vi "Timing FGV.vi"(8 "error in (no error)":errorcluster, 9 "Target time (s)":dbl format="%#_13g", 10 "Index":i32, 11 "Method (Get Time)":enum16{"Start", "Stop", "Reset", "Get Time"}(ring)=enum."Get Time") -> (0 "error out":errorcluster, 2 "Done":bool, 3 "Time Remaining(s)":dbl)   [LabVIEW 2013]
panel:
  out "Running":bool
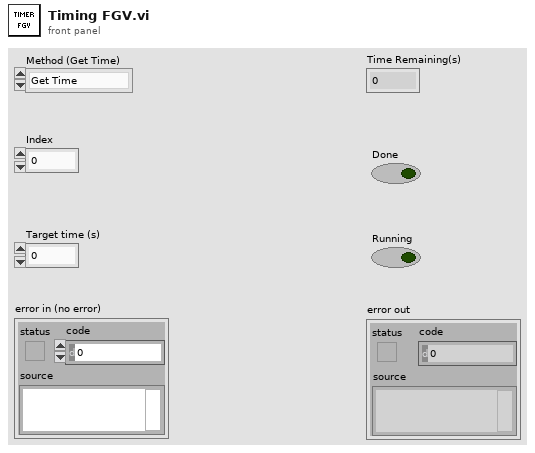
[diagram p1: front panel]
types:
  T1 = cluster{"Start Time":dbl, "Time Remaining":dbl, "Running":bool, "Done":bool}
  T2 = cluster{"Start Time":dbl, "Time Remaining":dbl, "Running":bool, "Done":bool}[]
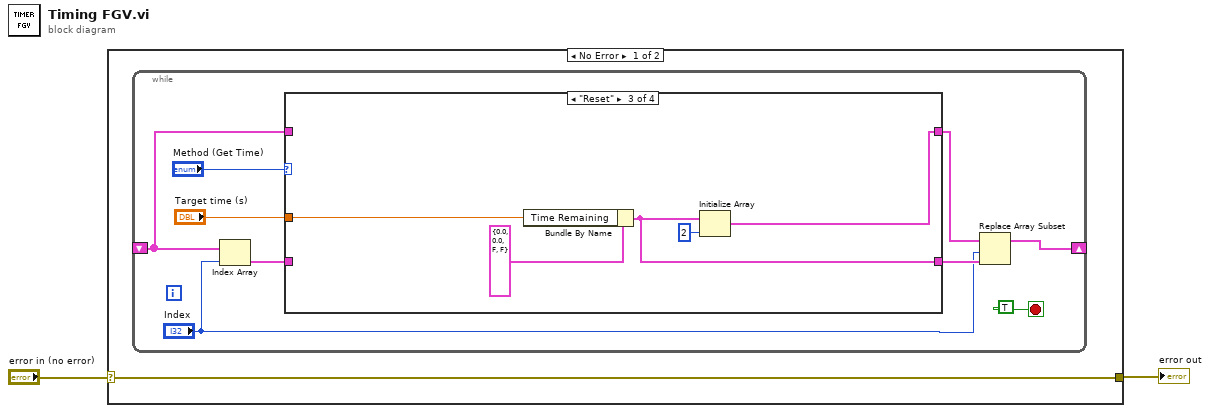
[diagram p0: block diagram]
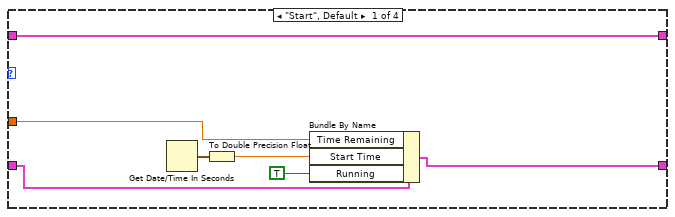
[diagram p2: hidden frame]
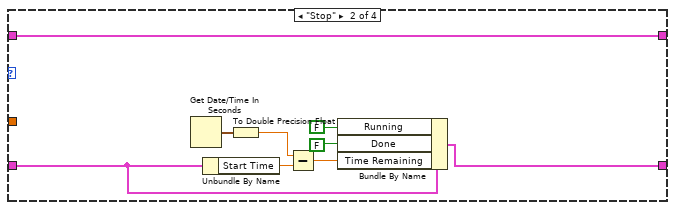
[diagram p3: hidden frame]
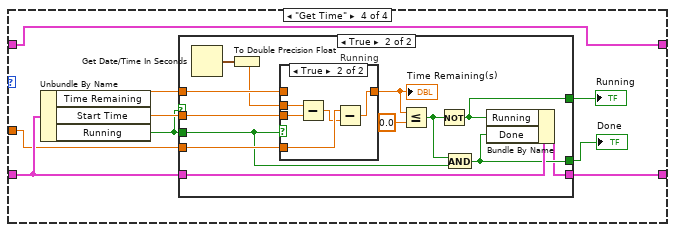
[diagram p4: hidden frame]
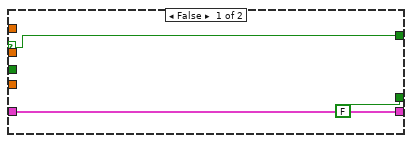
[diagram p5: hidden frame]
diagram:
  n1 = case shown="No Error" "error in (no error)" {
    selector: "error in (no error)" -> [w3 w65]
    tunnel: [w3 w65] -> w1
    frame No Error {
      n2 = while {
        shift-right: [w9] -> _
        shift-left: _ -> [w5]
        stop <- TRUE stop-if-true
        n3 = Index Array(array=w5, index="Index") -> (element=w7:T1)
        n4 = case shown="\"Reset\"" "Method (Get Time)" {
          tunnel: [w13 w22 w29 w36] -> w10
          tunnel: w7 -> [w18 w26 _ w40]
          tunnel: "Target time (s)" -> [w16 _ w32 w39]
          tunnel: w5 -> [w14 w23 _ w37]
          tunnel: [w14 w23 w30 w37] -> w4
          frame "Start", Default {
            n5 = Get Date/Time In Seconds() -> (seconds since 1Jan1904=w17:timestamp)
            n6 = To Double Precision Float(number=w17) -> (double precision float=w15:dbl)
            n7 = Bundle By Name(cluster=w18, "Time Remaining"=w16, "Start Time"=w15, "Running"=TRUE) -> (w13:T1)
          }
          frame "Stop" {
            n8 = Get Date/Time In Seconds() -> (seconds since 1Jan1904=w25:timestamp)
            n9 = Unbundle By Name(w26) -> ("Start Time"=w27:dbl)
            n10 = To Double Precision Float(number=w25) -> (double precision float=w24:dbl)
            n11 = Subtract(x=w24, y=w27) -> (x-y=w28:dbl)
            n12 = Bundle By Name(cluster=w26, "Running"=FALSE ("Done"), "Done"=FALSE, "Time Remaining"=w28) -> (w22:T1)
          }
          frame "Reset" {
            n13 = Bundle By Name(cluster=T1 {"Start Time"=0.0, "Time Remaining"=0.0, "Running"=FALSE, "Done"=FALSE}, "Time Remaining"=w32) -> (w29:T1)
            n14 = Initialize Array(w29, 2 ("dimension size")) -> (w30:T2)
          }
          frame "Get Time" {
            n15 = Unbundle By Name(w40) -> ("Time Remaining"=w42:dbl, "Start Time"=w41:dbl, "Running"=w35:bool)
            n16 = case shown="True" w35 {
              selector: w35 -> [w43 _]
              tunnel: w42 -> [_ w58]
              tunnel: w41 -> [_ w57]
              tunnel: w40 -> [w45 w54]
              tunnel: w39 -> [_ w53]
              tunnel: [FALSE w51] -> w38
              tunnel: [w45 w48] -> w36
              tunnel: w35 -> [_ w47]
              tunnel: [w43 w46] -> w34
              frame False {
              }
              frame True {
                n17 = Get Date/Time In Seconds() -> (seconds since 1Jan1904=w56:timestamp)
                n18 = To Double Precision Float(number=w56) -> (double precision float=w55:dbl)
                n19 = case "Running" shown="True" w47 {
                  tunnel: w55 -> [_ w64]
                  tunnel: w57 -> [_ w63]
                  tunnel: [w59 w62] -> w50
                  tunnel: w58 -> [w59 _]
                  tunnel: w53 -> [_ w61]
                  frame False {
                  }
                  frame True {
                    n20 = Subtract(x=w64, y=w63) -> (x-y=w60:dbl)
                    n21 = Subtract(x=w61, y=w60) -> (x-y=w62:dbl)
                  }
                }
                "Time Remaining(s)" <- w50
                n22 = Less Or Equal?(x=w50, y=0.0) -> (x <= y?=w52:bool)
                n23 = Not(x=w52) -> (.not. x?=w46:bool)
                n24 = And(x=w52, y=w47) -> (x .and. y?=w51:bool)
                n25 = Bundle By Name(cluster=w54, "Running"=w46, "Done"=w51) -> (w48:T1)
              }
            }
            "Running" <- w34
            "Done" <- w38
          }
        }
        n26 = Replace Array Subset(array=w4, new element=w10, index="Index") -> (w9:T2)
      }
    }
    frame Error {
    }
  }
  "error out" <- w1
